vi "main.vi"() -> ()   [LabVIEW 2014]
uses:
  <vilib>/Instr/_visa.llb/VISA Configure Serial Port (Instr).vi
panel:
  out "Seconds":sgl
  out "Chamber *C Data":string
  in  "Chamber *C Data":path=path "C:/Users/Administrator/Documents/humidity_sensing_setup/data/dumb/chamber_c_data.txt"
  out "Chamber *C Graph":sgl(graph)=5460.51
  out "Chamber *C":sgl
  out "Thermocouple Temperature Graph":sgl(graph)=5460.51
  out "Thermocouple Temperature":sgl
  out "Thermocouple *C Data":string
  in  "Thermocouple *C Data":path=path "C:/Users/Administrator/Documents/humidity_sensing_setup/data/dumb/thermocouple_c_data.txt"
  out "Pressure Data":string
  in  "Pressure Data":path=path "C:/Users/Administrator/Documents/humidity_sensing_setup/data/dumb/pressure_data.txt"
  out "Pressure Graph":sgl(graph)=5460.51
  out "Pressure":sgl
  in  "Start Button":bool
  out "Humidity":sgl
  out "Humidity Data":string
  in  "Humidity Data":path=path "C:/Users/Administrator/Documents/humidity_sensing_setup/data/dumb/humidity_data.txt"
  out "Humidity Data Graph":sgl(graph)=5460.51
  in  "Sampling rate (ms/pt)":i32=1000
  in  "stop button":bool
  in  "loop num":dbl=10000000000.0
  out "Arduino Status":bool
  out "error out":errorcluster
  in  "error in":errorcluster
  in  "instr name":string="Arduino"
  in  "write":bool
  in  "buffer size":u32=256
  in  "timeout (ms)":u32=10000
  in  "flow control":u16
  in  "stop bits":u16=10
  in  "parity":u16(ring) items=["None", "Odd", "Even", "Mark", "Space"]
  in  "data bits":u16=8 min=5 max=8 step=1
  in  "baud rate":u32=9600
  in  "write string":string
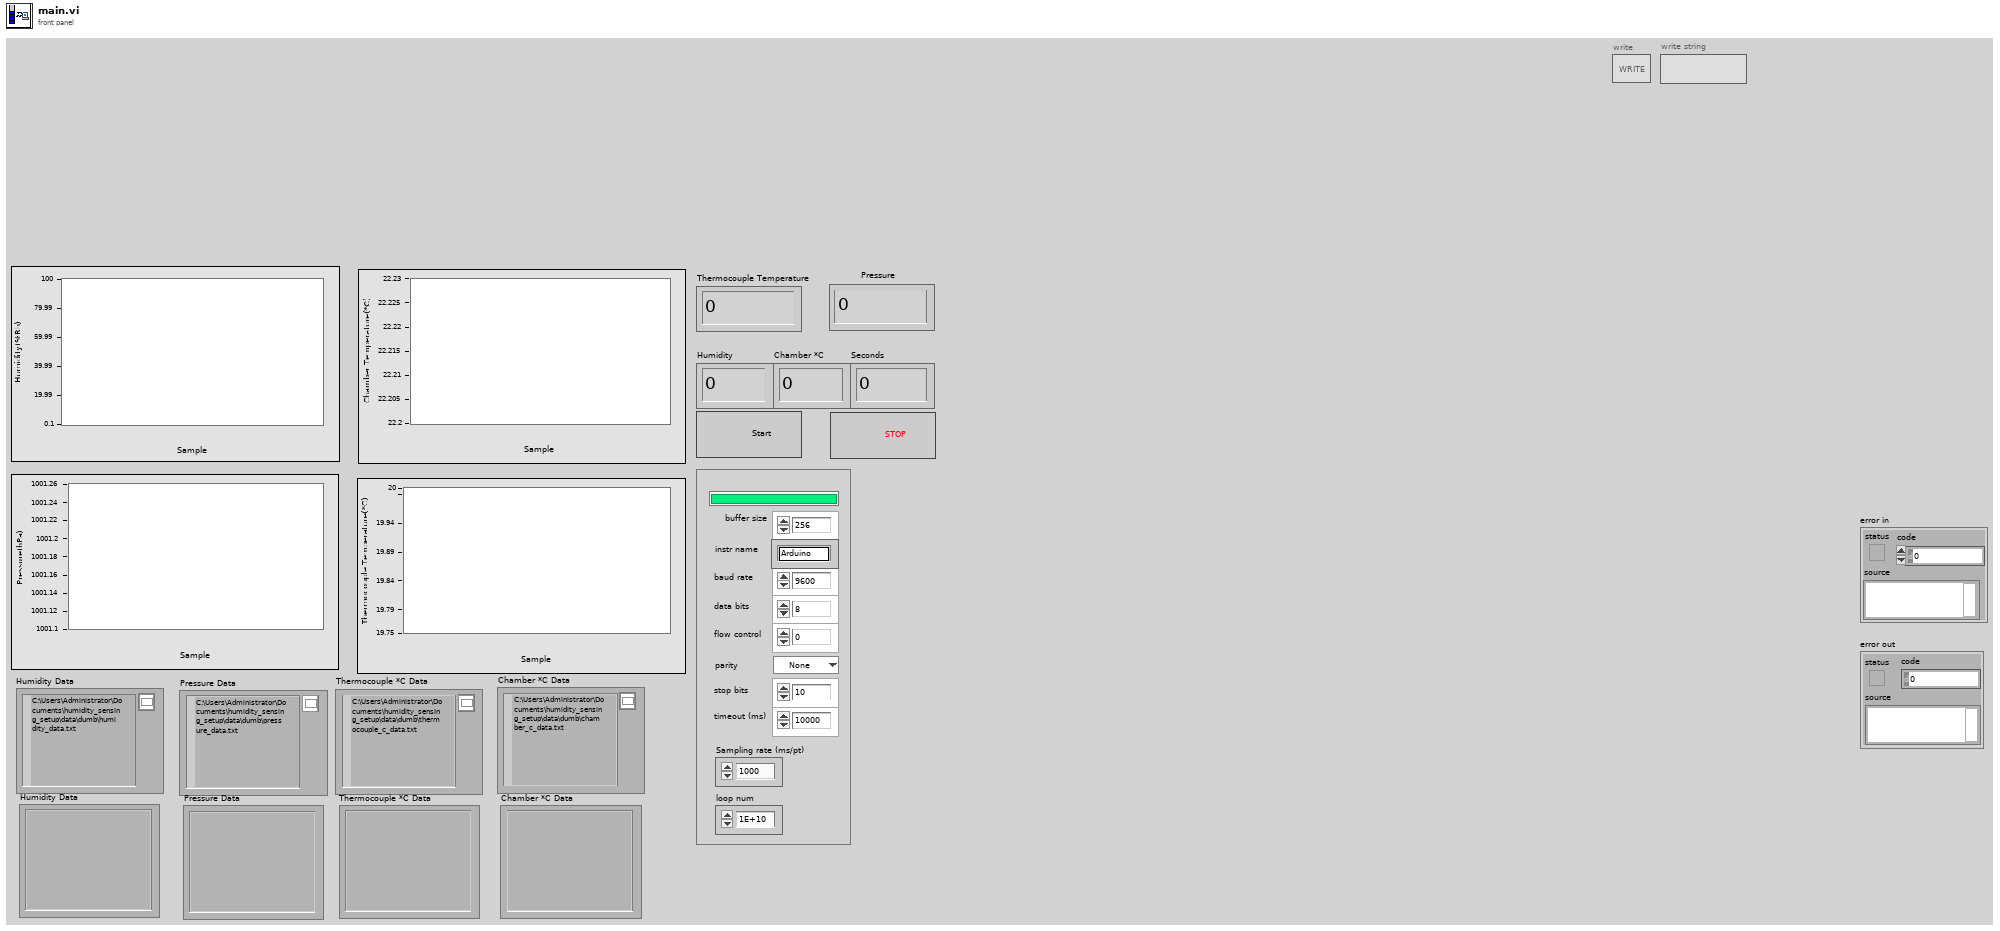
[diagram p1: front panel]
types:
  T1 = enum16{"open", "replace", "create", "open or create", "replace or create", "replace or create with confirmation"}
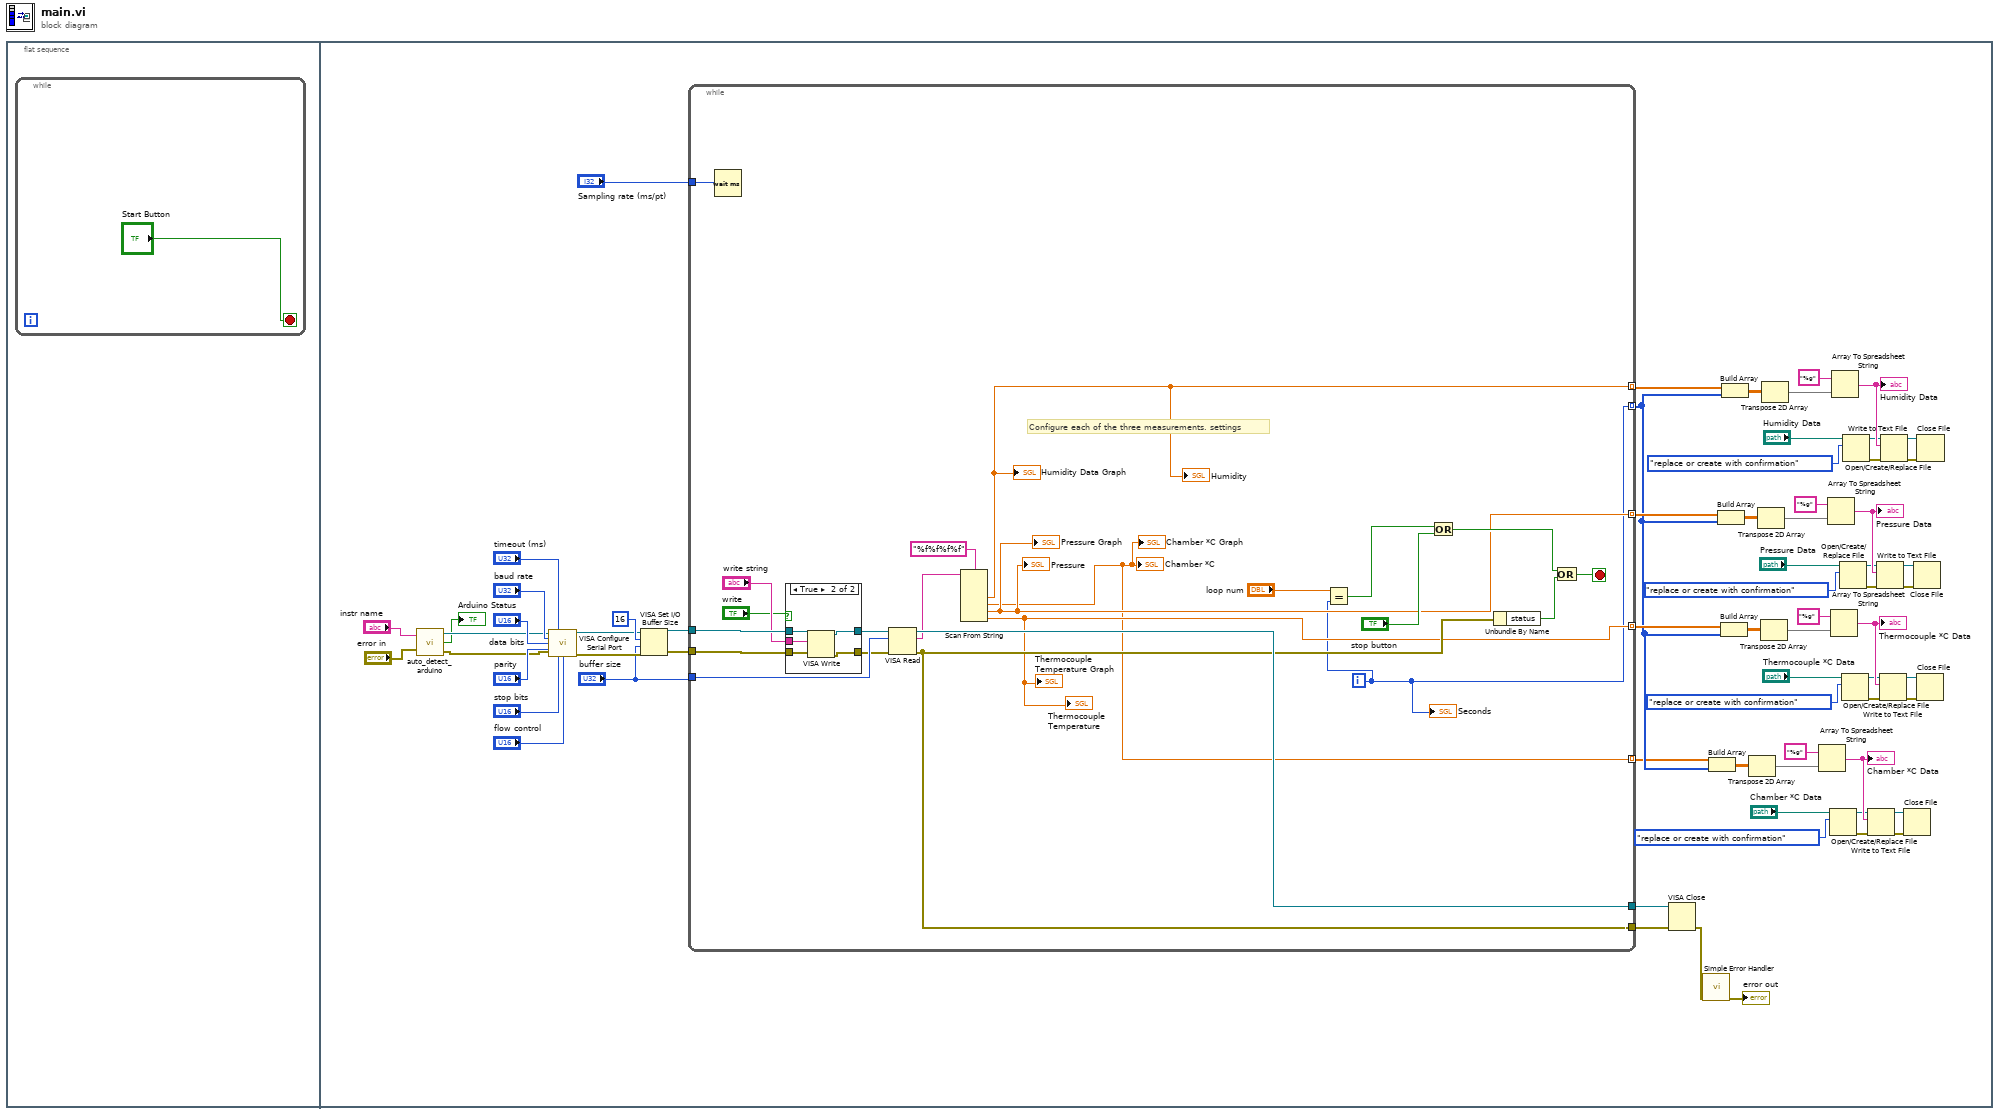
[diagram p0: block diagram]
diagram:
  n1 = flat-sequence {
    frame #0 {
      n2 = while {
        stop <- "Start Button" stop-if-true
      }
    }
    frame #1 {
      n3 = call "auto_detect_arduino.vi"("instr name"="instr name", "error in"="error in") -> ("VISA resource name"=w60:refnum<visa-resource-name>, "status"=→"Arduino Status":bool, "error out"=w59:errorcluster)
      n4 = call-poly "VISA Configure Serial Port"("VISA resource name"=w60, "timeout (10sec)"="timeout (ms)", "baud rate (9600)"="baud rate", "data bits (8)"="data bits", "parity (0:none)"="parity", "error in (no error)"=w59, "stop bits (10: 1 bit)"="stop bits", "flow control (0:none)"="flow control") -> ("VISA resource name out"=w56:refnum<visa-resource-name>, "error out"=w55:errorcluster)  [unwired: 6 in]
      n5 = VISA Set I/O Buffer Size(VISA resource name=w56, mask (16)=u16 16 ("I/O Receive\nBuffer mask"), size (4096)="buffer size", error in (no error)=w55) -> (VISA resource name out=w54:refnum<visa-resource-name>, error out=w53:errorcluster)
      n6 = while {
        tunnel: w54 -> [w88]
        tunnel: w53 -> [w87]
        tunnel: [w89] -> w68
        tunnel: [w77] -> w67
        tunnel: "buffer size" -> [w90]
        tunnel: [w78] -> w36 mode=indexing
        tunnel: "Sampling rate (ms/pt)" -> [w80]
        tunnel: [w70] -> w3 mode=indexing
        tunnel: [w73] -> w25 mode=indexing
        tunnel: [w72] -> w14 mode=indexing
        tunnel: [w71] -> w2 mode=indexing
        i -> [w70]
        stop <- w91 stop-if-true
        # "Configure each of the three measurements. settings"
        n7 = Wait (ms)(milliseconds to wait=w80) -> ()  [unwired: 1 out]
        n8 = case shown="True" "write" {
          tunnel: w88 -> [w93 w98]
          tunnel: w87 -> [w92 w97]
          tunnel: [w93 w96] -> w86
          tunnel: [w92 w95] -> w85
          tunnel: "write string" -> [_ w94]
          frame False {
          }
          frame True {
            n9 = VISA Write(VISA resource name=w98, write buffer=w94, error in (no error)=w97) -> (VISA resource name out=w96:refnum<visa-resource-name>, error out=w95:errorcluster)  [unwired: 1 out]
          }
        }
        n10 = VISA Read(VISA resource name=w86, byte count=w90, error in (no error)=w85) -> (VISA resource name out=w89:refnum<visa-resource-name>, read buffer=w74:string, error out=w77:errorcluster)  [unwired: 1 out]
        n11 = Scan From String(format string="%f%f%f%f", input string=w74) -> (output 1=w78:sgl, output 2=w71:sgl, output 3=w73:sgl, output 4=w72:sgl)  [unwired: 6 in, 3 out]
        "Humidity Data Graph" <- w78
        "Humidity" <- w78
        "Pressure" <- w73
        "Pressure Graph" <- w73
        "Thermocouple Temperature" <- w72
        "Thermocouple Temperature Graph" <- w72
        "Chamber *C" <- w71
        "Chamber *C Graph" <- w71
        n12 = Equal?(x="loop num", y=w70) -> (x = y?=w69:bool)
        n13 = Or(x=w69, y="stop button") -> (x .or. y?=w75:bool)
        n14 = Unbundle By Name(w77) -> ("status"=w76:bool)
        n15 = Or(x=w75, y=w76) -> (x .or. y?=w91:bool)
        "Seconds" <- w70
      }
      n16 = VISA Close(VISA resource name=w68, error in (no error)=w67) -> (error out=w50:errorcluster)
      n17 = call <vilib>:"Simple Error Handler.vi"("error in (no error)"=w50) -> ("error out"=→"error out":errorcluster)  [unwired: 4 in, 4 out]
      n18 = Build Array(w2, w3) -> (w4:sgl[][])
      n19 = Build Array(w25, w3) -> (w26:sgl[][])
      n20 = Build Array(w14, w3) -> (w15:sgl[][])
      n21 = Build Array(w36, w3) -> (w37:sgl[][])
      n22 = Transpose 2D Array(2D array=w4) -> (transposed array=w12:sgl[][])
      n23 = Transpose 2D Array(2D array=w26) -> (transposed array=w34:sgl[][])
      n24 = Transpose 2D Array(2D array=w15) -> (transposed array=w23:sgl[][])
      n25 = Transpose 2D Array(2D array=w37) -> (transposed array=w45:sgl[][])
      n26 = Array To Spreadsheet String(array=w12, 3:"%g" ("format string")) -> (spreadsheet string=w13:string)  [unwired: 1 in]
      "Chamber *C Data" <- w13
      n27 = Array To Spreadsheet String(array=w34, 3:"%g" ("format string")) -> (spreadsheet string=w35:string)  [unwired: 1 in]
      "Pressure Data" <- w35
      n28 = Open/Create/Replace File(file path (use dialog)="Chamber *C Data", operation (0:open)=T1."replace or create with confirmation") -> (refnum out=w10:refnum<file>, error out=w5:errorcluster)  [unwired: 4 in, 1 out]
      n29 = Array To Spreadsheet String(array=w23, 3:"%g" ("format string")) -> (spreadsheet string=w24:string)  [unwired: 1 in]
      "Thermocouple *C Data" <- w24
      n30 = Array To Spreadsheet String(array=w45, 3:"%g" ("format string")) -> (spreadsheet string=w46:string)  [unwired: 1 in]
      "Humidity Data" <- w46
      n31 = Open/Create/Replace File(file path (use dialog)="Pressure Data", operation (0:open)=T1."replace or create with confirmation") -> (refnum out=w32:refnum<file>, error out=w27:errorcluster)  [unwired: 4 in, 1 out]
      n32 = Open/Create/Replace File(file path (use dialog)="Thermocouple *C Data", operation (0:open)=T1."replace or create with confirmation") -> (refnum out=w21:refnum<file>, error out=w16:errorcluster)  [unwired: 4 in, 1 out]
      n33 = Open/Create/Replace File(file path (use dialog)="Humidity Data", operation (0:open)=T1."replace or create with confirmation") -> (refnum out=w43:refnum<file>, error out=w38:errorcluster)  [unwired: 4 in, 1 out]
      n34 = Write to Text File(file (use dialog)=w10, text=w13, error in=w5) -> (refnum out=w7:refnum<file>, error out=w6:errorcluster)  [unwired: 2 out]
      n35 = Write to Text File(file (use dialog)=w32, text=w35, error in=w27) -> (refnum out=w29:refnum<file>, error out=w28:errorcluster)  [unwired: 2 out]
      n36 = Write to Text File(file (use dialog)=w21, text=w24, error in=w16) -> (refnum out=w18:refnum<file>, error out=w17:errorcluster)  [unwired: 2 out]
      n37 = Write to Text File(file (use dialog)=w43, text=w46, error in=w38) -> (refnum out=w40:refnum<file>, error out=w39:errorcluster)  [unwired: 2 out]
      n38 = Close File(refnum=w7, error in=w6) -> ()  [unwired: 2 out]
      n39 = Close File(refnum=w29, error in=w28) -> ()  [unwired: 2 out]
      n40 = Close File(refnum=w18, error in=w17) -> ()  [unwired: 2 out]
      n41 = Close File(refnum=w40, error in=w39) -> ()  [unwired: 2 out]
    }
  }
